vi "Launch Piston Heater.vi"(8 "error in (no error)":errorcluster, 11 "cRIO-CO2 in":refnum<class "cRIO-CO2.lvclass">) -> (0 "error out":errorcluster, 3 "cRIO-CO2 out":refnum<class "cRIO-CO2.lvclass">)   [LabVIEW 2015, in "cRIO-Carbondioxide.lvlib" / "cRIO-CO2.lvlib" / "cRIO-CO2.lvclass"]
uses:
  cRIO-CO2.lvclass
  cRIO-CO2.lvclass/cRIO-CO2.ctl
  CO2 Actor Messages/Ping Msg/Ping Msg.lvclass/Ping Msg.ctl
  <vilib>/ActorFramework/Message Enqueuer/Message Enqueuer.lvclass/Message Enqueuer.ctl
  cRIO-CO2 Messages/Log Message Msg/Log Message Msg.lvclass/Log Message Msg.ctl
  <vilib>/ActorFramework/Message Enqueuer/Enqueue.vi
  <vilib>/ActorFramework/Message Priority Queue/Priority Enqueue.vi
  CO2 Actor Messages/Ping Msg/Ping Msg.lvclass
  <vilib>/ActorFramework/Actor/Actor.lvclass
  cRIO-CO2 Messages/Log Message Msg/Log Message Msg.lvclass
  <vilib>/ActorFramework/Message Enqueuer/Message Enqueuer.lvclass
  Heater/Heater.lvclass
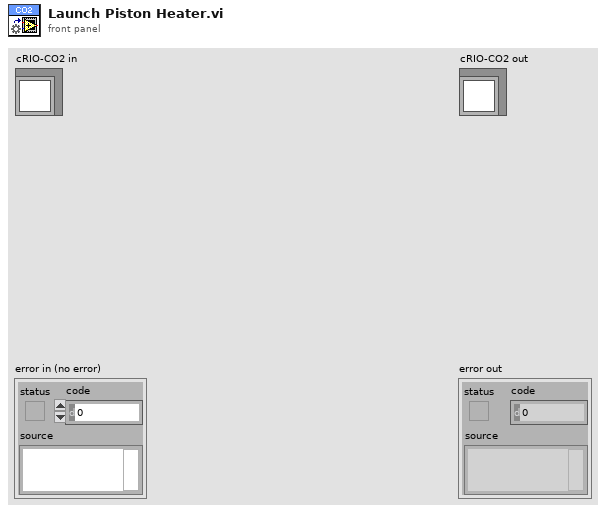
[diagram p1: front panel]
types:
  T1 = cluster{"Heater Duty Cycle SHV":refnum<k21>, "Thermocouple SHV":refnum<k21>, "Setpoint SHV":refnum<k21>, "Switch SHV":refnum<k21>}
  T2 = cluster{"PID":cluster{"P":dbl, "I":dbl, "D":dbl}, "Upper Limit":dbl, "Lower Limit":dbl}
  T3 = typedef "Dedicated Enqueuers.ctl" = cluster{"Freezers":cluster{"Syringe":refnum<class "Message Enqueuer.lvclass">, "Tank 1":refnum<class "Message Enqueuer.lvclass">, "Tank 2":refnum<class "Message Enqueuer.lvclass">, "Tank 3":refnum<class "Message Enqueuer.lvclass">, "Tank 4":refnum<class "Message Enqueuer.lvclass">}, "Heaters":cluster{"Syringe":refnum<class "Message Enqueuer.lvclass">, "Piston":refnum<class "Message Enqueuer.lvclass">}, "Blowers":cluster{"Tank 1":refnum<class "Message Enqueuer.lvclass">, "Tank 2":refnum<class "Message Enqueuer.lvclass">, "Tank 3":refnum<class "Message Enqueuer.lvclass">, "Tank 4":refnum<class "Message Enqueuer.lvclass">, "Syringe":refnum<class "Message Enqueuer.lvclass">}, "Sample Line":refnum<class "Message Enqueuer.lvclass">, "Storage Line":refnum<class "Message Enqueuer.lvclass">, "Transfer Line":refnum<class "Message Enqueuer.lvclass">, "Syringe Stepper":refnum<class "Message Enqueuer.lvclass">, "Syringe Line":refnum<class "Message Enqueuer.lvclass">, "Capillary Line":refnum<class "Message Enqueuer.lvclass">, "Preparation Line":refnum<class "Message Enqueuer.lvclass">, "Turbo":refnum<class "Message Enqueuer.lvclass">, "Vacuum":refnum<class "Message Enqueuer.lvclass">, "He Line":refnum<class "Message Enqueuer.lvclass">, "Cylinder":refnum<class "Message Enqueuer.lvclass">}
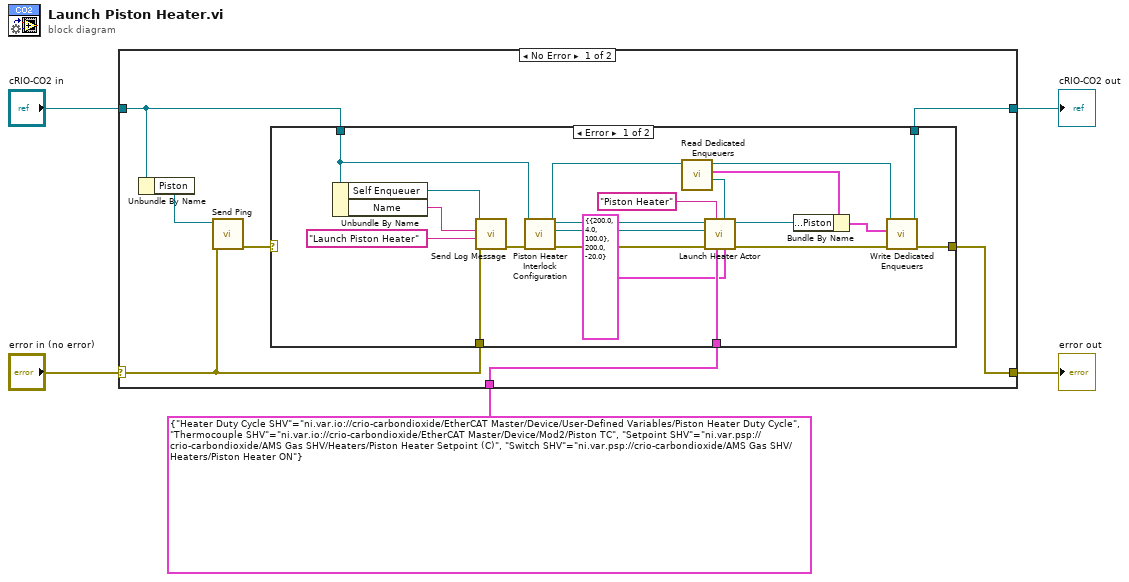
[diagram p0: block diagram]
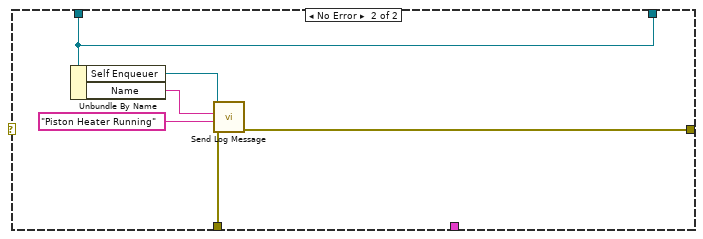
[diagram p2: hidden frame]
diagram:
  n1 = case shown="No Error" "error in (no error)" {
    selector: "error in (no error)" -> [w10 w40]
    tunnel: [w6 w40] -> w4
    tunnel: [w8 w39] -> w2
    tunnel: "cRIO-CO2 in" -> [w11 w39]
    tunnel: T1 {"Heater Duty Cycle SHV"="ni.var.io://crio-carbondioxide/EtherCAT Master/Device/User-Defined Variables/Piston Heater Duty Cycle", "Thermocouple SHV"="ni.var.io://crio-carbondioxide/EtherCAT Master/Device/Mod2/Piston TC", "Setpoint SHV"="ni.var.psp://crio-carbondioxide/AMS Gas SHV/Heaters/Piston Heater Setpoint (C)", "Switch SHV"="ni.var.psp://crio-carbondioxide/AMS Gas SHV/Heaters/Piston Heater ON"} -> [w12 _]
    frame No Error {
      n2 = Unbundle By Name(w11) -> ("Piston"=w7:refnum<class "Message Enqueuer.lvclass">)
      n3 = call "Send Ping.vi"("error in (no error)"=w10, "Message Enqueuer"=w7) -> ("error out"=w9:errorcluster)  [unwired: 6 in, 3 out]
      n4 = case shown="Error" w9 {
        tunnel: w12 -> [w25 _]
        tunnel: w11 -> [w23 w34]
        tunnel: w10 -> [w24 w35]
        tunnel: [w20 w34] -> w8
        tunnel: [w19 w33] -> w6
        frame Error {
          n5 = Unbundle By Name(w23) -> ("Self Enqueuer"=w29:refnum<class "Message Enqueuer.lvclass">, "Name"=w31:string)
          n6 = call "Send Log Message.vi"("error in (no error)"=w24, "String"="Launch Piston Heater", "Source Name"=w31, "Message Enqueuer"=w29) -> ("error out"=w28:errorcluster)  [unwired: 6 in, 1 out]
          n7 = call "Piston Heater Interlock Configuration.vi"("error in (no error)"=w28, "cRIO-CO2 in"=w23) -> ("error out"=w26:errorcluster, "Interlock Chain"=w27:refnum<class "Interlock Chain.lvclass">, "cRIO-CO2 out"=w18:refnum<class "cRIO-CO2.lvclass">)  [unwired: 7 in]
          n8 = call "Read Dedicated Enqueuers.vi"("cRIO-CO2 in"=w18) -> ("Qs.DedicatedEnQrs"=w15:refnum<queue>, "Dedicated Enqueuers"=w22:T3, "cRIO-CO2 out"=w14:refnum<class "cRIO-CO2.lvclass">)  [unwired: 7 in, 1 out]
          n9 = call "Launch Heater Actor.vi"("PID."=T2 {"PID"={"P"=200.0, "I"=4.0, "D"=100.0}, "Upper Limit"=200.0, "Lower Limit"=-20.0}, "DedicatedEnQrs"=w15, "SHVs"=w25, "Name"="Piston Heater", "error in (no error)"=w26, "Interlock Chain"=w27, "Caller Actor in"=w18) -> ("error out"=w16:errorcluster, "Caller-To-Actor Enqueuer"=w21:refnum<class "Message Enqueuer.lvclass">)  [unwired: 3 in]
          n10 = Bundle By Name(cluster=w22, "Heaters.Piston"=w21) -> (w13:T3)
          n11 = call "Write Dedicated Enqueuers.vi"("error in (no error)"=w16, "Dedicated Enqueuers"=w13, "cRIO-CO2 in"=w14) -> ("error out"=w19:errorcluster, "cRIO-CO2 out"=w20:refnum<class "cRIO-CO2.lvclass">)  [unwired: 7 in]
        }
        frame No Error {
          n12 = Unbundle By Name(w34) -> ("Self Enqueuer"=w36:refnum<class "Message Enqueuer.lvclass">, "Name"=w38:string)
          n13 = call "Send Log Message.vi"("error in (no error)"=w35, "String"="Piston Heater Running", "Source Name"=w38, "Message Enqueuer"=w36) -> ("error out"=w33:errorcluster)  [unwired: 6 in, 1 out]
        }
      }
    }
    frame Error {
    }
  }
  "error out" <- w4
  "cRIO-CO2 out" <- w2
